vi "1-15.vi"() -> ()   [LabVIEW 2022 SP3]
panel:
  out "S":dbl
  out "X":dbl
  in  "M":dbl
  in  "N":dbl
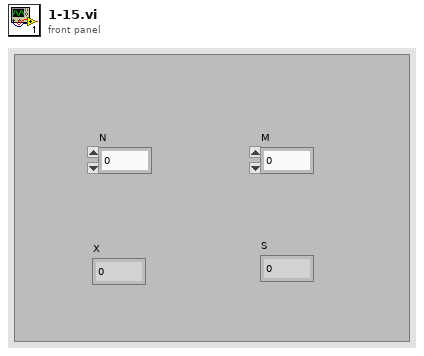
[diagram p1: front panel]
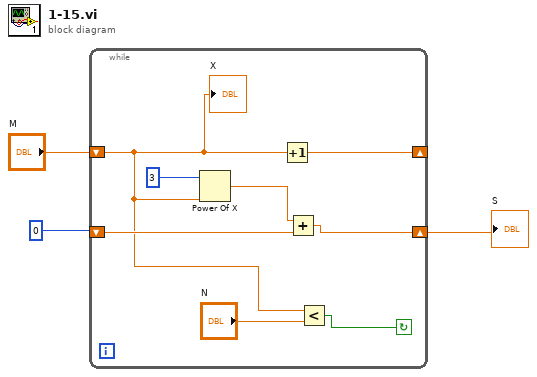
[diagram p0: block diagram]
diagram:
  n1 = while {
    shift-right: [w7] -> _
    shift-left: "M" -> [w4]
    shift-right: [w10] -> w1
    shift-left: 0 -> [w11]
    stop <- w5 continue-if-true
    n2 = Power Of X(1:w4, 2:3) -> (0:w9:dbl)
    n3 = Increment(x=w4) -> (x+1=w7:dbl)
    n4 = Add(x=w9, y=w11) -> (x+y=w10:dbl)
    n5 = Less?(x=w4, y="N") -> (x < y?=w5:bool)
    "X" <- w4
  }
  "S" <- w1
